vi "Test Open IPS.vi"(8 "error in (no error)":errorcluster, 11 "Instrument.OxfordVRM in":refnum<class "Instrument.OxfordVRM.lvclass">) -> (0 "error out":errorcluster, 3 "Instrument.OxfordVRM out":refnum<class "Instrument.OxfordVRM.lvclass">)   [LabVIEW 2019, in "Instrument.OxfordVRM.lvclass"]
uses:
  Instrument.OxfordVRM.lvclass
  <vilib>/addons/_JKI Toolkits/Caraya/classes/Assert/Assert.lvclass
  <instrlib>/Mercury iXX/Public/Controls/Comms Transport Layer.ctl
  <instrlib>/Mercury iXX/Mercury iXX.lvlib
  <instrlib>/Mercury iXX/Private/Controls/Query Dynamic Reference.ctl
  <instrlib>/Mercury iXX/Public/Controls/Mercury Reference.ctl
  <vilib>/addons/_JKI Toolkits/Caraya/classes/Test/Test.lvclass
  <vilib>/addons/_JKI Toolkits/Caraya/classes/Assert/Assert Not Error.vi
  <vilib>/addons/_JKI Toolkits/Caraya/classes/Assert/Assert Not Equal Value_Variant.vi
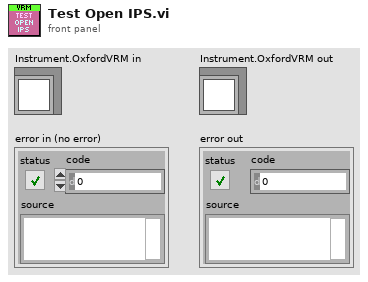
[diagram p1: front panel]
types:
  T1 = typedef "Mercury iXX.lvlib/Mercury Reference.ctl" = cluster{"Comms":refnum<visa-resource-name>, "Device ID":string[], "Comms Layer":T2, "Command":string, "Query reference":T3}
  T2 = typedef "Mercury iXX.lvlib/Comms Transport Layer.ctl" = enum16{"Ethernet TCP/IP", "USB", "ISOBus - RS-232", "GPIB"}
  T3 = typedef "Mercury iXX.lvlib/Query Dynamic Reference.ctl" = refnum<vi>
  T4 = cluster{"Address":string, "Reference":T1, "Devices":cluster{"Temperature":string, "Magnet X":string, "Magnet Y":string, "Magnet Z":string, "PSU 1":string, "PSU 2":string, "PSU 3":string, "PSU 4":string, "PSU 5":string, "PSU 6":string}}
  T5 = cluster{"Reference":T1, "Devices":cluster{"Temperature":string, "Magnet X":string, "Magnet Y":string, "Magnet Z":string, "PSU 1":string, "PSU 2":string, "PSU 3":string, "PSU 4":string, "PSU 5":string, "PSU 6":string}}
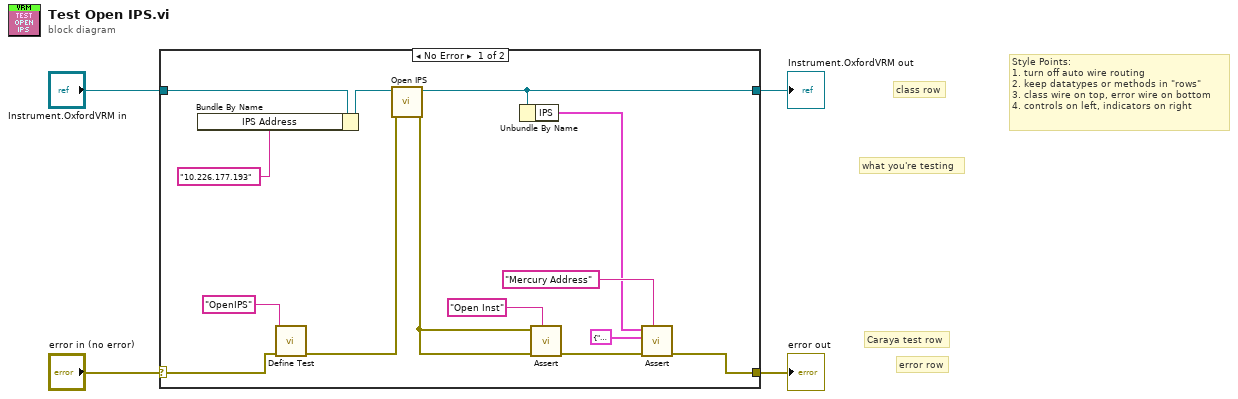
[diagram p0: block diagram]
diagram:
  # "what you're testing"
  # "Caraya test row"
  # "error row"
  # "class row"
  # "Style Points:\n1. turn off auto wire routing\n2. keep datatypes or methods in \"rows\"\n3. class wire on top, error wire on bottom\n4. controls on left, indicators on right"
  n1 = case shown="No Error" "error in (no error)" {
    selector: "error in (no error)" -> [w9 w20]
    tunnel: [w8 w20] -> w1
    tunnel: [w5 w19] -> w2
    tunnel: "Instrument.OxfordVRM in" -> [w6 w19]
    frame No Error {
      n2 = Bundle By Name(cluster=w6, "IPS Address"="10.226.177.193" ("IP Address")) -> (w7:refnum<class "Instrument.OxfordVRM.lvclass">)
      n3 = call <vilib>:"Define Test.vi"("error in (no error)"=w9, "Label (VI Title)"="OpenIPS") -> ("error out"=w15:errorcluster)  [unwired: 8 in, 1 out]
      n4 = call "Open IPS.vi"("error in (no error)"=w15, "Instrument.OxfordVRM in"=w7) -> ("error out"=w16:errorcluster, "Instrument.OxfordVRM out"=w5:refnum<class "Instrument.OxfordVRM.lvclass">)  [unwired: 8 in]
      n5 = Unbundle By Name(w5) -> ("IPS"=w11:T5)
      n6 = call-poly <vilib>:"Assert.vi"("Label"="Open Inst", "error in (no error)"=w16, "Not Error?"=w16) -> ("error out"=w13:errorcluster)  [unwired: 7 in, 1 out]
      n7 = call-poly <vilib>:"Assert.vi"("Label"="Mercury Address", "error in (no error)"=w13, "Y"=T4 {"Address"="", "Reference"={"Comms"="", "Device ID"=[], "Comms Layer"=enum."Ethernet TCP/IP", "Command"="", "Query reference"=refnum}, "Devices"={"Temperature"="", "Magnet X"="", "Magnet Y"="", "Magnet Z"="", "PSU 1"="", "PSU 2"="", "PSU 3"="", "PSU 4"="", "PSU 5"="", "PSU 6"=""}} ("IPS"), "X"=w11) -> ("error out"=w8:errorcluster)  [unwired: 6 in, 1 out]
    }
    frame Error {
    }
  }
  "error out" <- w1
  "Instrument.OxfordVRM out" <- w2
